vi "TagDB Refmgr-Refresh.vi"(0 "DB Ref":T1, 5 "StateName":string[](array[string]), 7 "State":i32[](array[numeric]), 9 "RulesMap":variant[](array[variant]), 11 "error in (no error)":errorcluster) -> (4 "DB Ref (dup)":T1, 15 "error out":errorcluster)   [LabVIEW 2017, in "TagDB UIStateExpression.lvlib"]
uses:
  TagDB UIStateExpression.lvlib
  <userlib>/_NEVSTOP/TagDB/Typedef/TagDB.ctl
  ffb2c392-d373-42eb-b860-446857515c6d.vi
  ef9e8651-8229-402e-944d-f981edee3a32.vi
  <userlib>/_NEVSTOP/TagDB/TagDB.lvlib
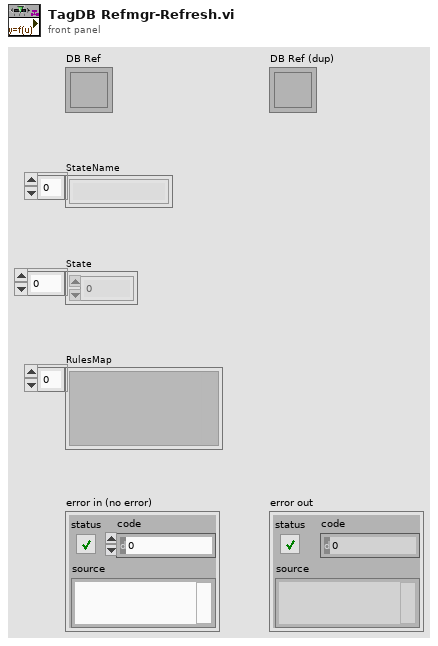
[diagram p1: front panel]
types:
  T1 = typedef "TagDB.lvlib/TagDB.ctl" = refnum<k1>
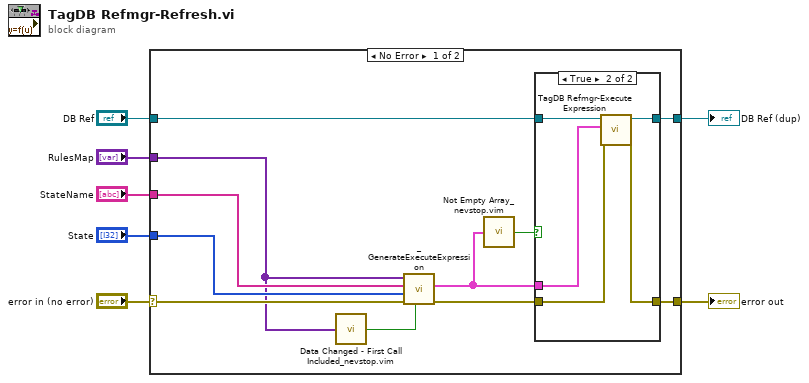
[diagram p0: block diagram]
diagram:
  n1 = case shown="No Error" "error in (no error)" {
    selector: "error in (no error)" -> [w14 w27]
    tunnel: [w16 w27] -> w6
    tunnel: "DB Ref" -> [w15 w26]
    tunnel: [w18 w26] -> w4
    tunnel: "RulesMap" -> [w11 _]
    tunnel: "StateName" -> [w13 _]
    tunnel: "State" -> [w12 _]
    frame No Error {
      n2 = call "Data Changed - First Call Included_nevstop.vim"("Variant"=w11) -> ("Changed"=w10:bool)
      n3 = call "_GenerateExecuteExpression.vi"("first call?"=w10, "error in (no error)"=w14, "States"=w12, "StateNames"=w13, "RulesMap"=w11) -> ("error out"=w17:errorcluster, "exps"=w9:cluster{"Tag":string, "formula":string}[])  [unwired: 4 in, 1 out]
      n4 = call "Not Empty Array_nevstop.vim"("Array"=w9) -> ("not empty?"=w8:bool)
      n5 = case shown="True" w8 {
        tunnel: [w19 w25] -> w18
        tunnel: w17 -> [w20 w24]
        tunnel: [w20 w23] -> w16
        tunnel: w15 -> [w19 w22]
        tunnel: w9 -> [_ w21]
        frame False {
        }
        frame True {
          n6 = call "TagDB Refmgr-Execute Expression.vi"("error in (no error)"=w24, "expressions"=w21, "DB Ref"=w22) -> ("error out"=w23:errorcluster, "DB Ref (dup)"=w25:T1)  [unwired: 6 in, 1 out]
        }
      }
    }
    frame Error {
    }
  }
  "error out" <- w6
  "DB Ref (dup)" <- w4
